vi "喂猫.vi"() -> (3 "数值":i8)   [LabVIEW 2011]
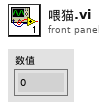
[diagram p1: front panel]
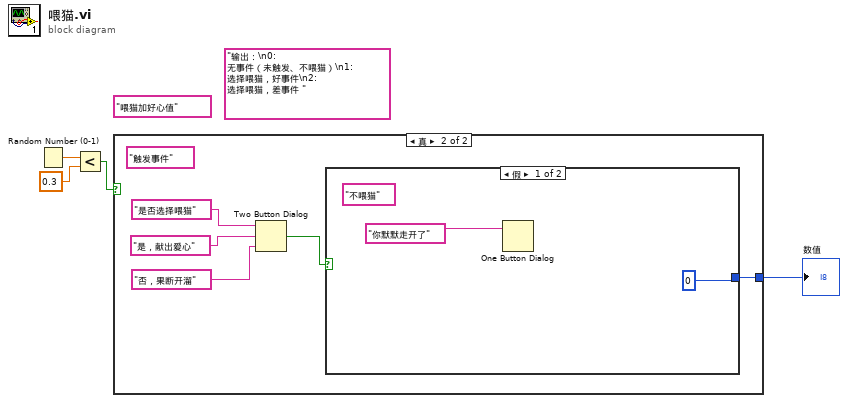
[diagram p0: block diagram]
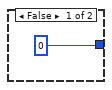
[diagram p2: hidden frame]
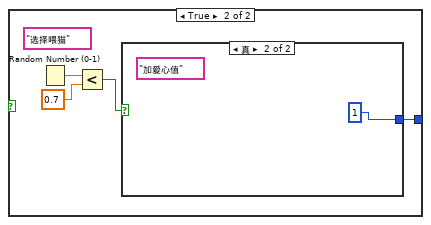
[diagram p3: hidden frame]
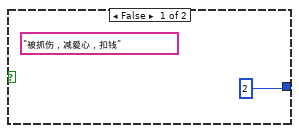
[diagram p4: hidden frame]
diagram:
  (unwired) "输出：\n0: 无事件（未触发、不喂猫）\n1: 选择喂猫，好事件\n2: 选择喂猫，差事件 "
  (unwired) "喂猫加好心值"
  n1 = Random Number (0-1)() -> (number: 0 to 1=w4:dbl)
  n2 = Less?(x=w4, y=0.3) -> (x < y?=w2:bool)
  n3 = case shown="真" w2 {
    tunnel: [0 w6] -> w1
    frame False {
    }
    frame True {
      (unwired) "触发事件"
      n4 = Two Button Dialog(message="是否选择喂猫", 1:"否，果断开溜", 2:"是，献出爱心") -> (T button?=w7:bool)
      n5 = case shown="假" w7 {
        tunnel: [0 w13] -> w6
        frame False {
          (unwired) "不喂猫"
          n6 = One Button Dialog(message="你默默走开了") -> ()  [unwired: 1 in, 1 out]
        }
        frame True {
          (unwired) "选择喂猫"
          n7 = Random Number (0-1)() -> (number: 0 to 1=w16:dbl)
          n8 = Less?(x=w16, y=0.7) -> (x < y?=w14:bool)
          n9 = case shown="真" w14 {
            tunnel: [2 1] -> w13
            frame False {
              (unwired) "被抓伤，减爱心，扣钱"
            }
            frame True {
              (unwired) "加爱心值"
            }
          }
        }
      }
    }
  }
  "数值" <- w1
